vi "Stop Core.vi"(10 "final error code":i32, 11 "Generador de Señales in":refnum<class "Generador de Señales.lvclass">) -> (3 "Generador de Señales out":refnum<class "Generador de Señales.lvclass">)   [LabVIEW 2020, in "Generador de Señales.lvlib" / "Generador de Señales.lvclass"]
doc: "(<B>Filename</B>: Actor Framework.lvlib:Actor.lvclass:Stop Core.vi)\n\nDefines what the actor does before it stops. Use the <B>final error code</B> input to determine whether the actor shut down in response to an error.\n\nBy default, this method passes the Stop message along to all auto-stop nested actors. A descendant class may override this method to define additional behavior, such as shutting down any processes the actor initiated in its override of the Actor Core method."
uses:
  <vilib>/ActorFramework/Actor/Actor.lvclass
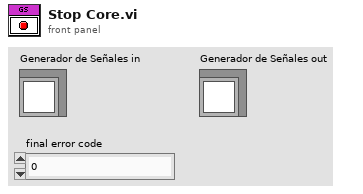
[diagram p1: front panel]
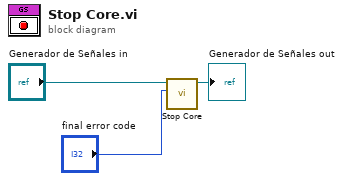
[diagram p0: block diagram]
diagram:
  n1 = call-parent "Stop Core.vi"("final error code"="final error code", "Actor in"="Generador de Señales in") -> ("Actor out"=→"Generador de Señales out":refnum<class "Generador de Señales.lvclass">)  [unwired: 9 in]
